vi "Open FPGA Reference.vi"(8 "Error In":errorcluster, 11 "Settings.Compiled":T18={"Name"="", "RIO.Address"="", "Bitfile.Path"=path "", "Injectors.Count"=0, "Injectors.Settings"=[], "Waveform.Refs"=[], "VS.Registers"={"Block Data refs"=[], "Values"=[]}, "Registers"=[], "Timing.Registers"=[], "Mux.Register"={"Name"="", "Data Type"=enum."<Null>", "Default Value"=variant(dbl 0.0)}, "Groups.Settings"=[]} {"Mux.Register"."Data Type" format="%.0x"; "Registers"."Register"."Data Type" format="%.0x"; "VS.Registers"."Block Data refs"."Data Reference" format="%.0x"}) -> (0 "Error Out":errorcluster, 2 "Async Parameters":T1, 3 "Inline State Data out":T13 {"VS.Registers"."Data Reference" format="%.0x"; "FPGA.Registers"."Data Type" format="%.0x"})   [LabVIEW 2019, in "Fuel Injector Analysis Addon Engine.lvlib"]
uses:
  Fuel Injector Analysis Addon Engine.lvlib
  Shared/Types/Compiled.Settings.ctl
  Shared/Types/Injector info.ctl
  Shared/Types/Compiled.Group.WaveformRefs.ctl
  <vilib>/NI VeriStand/Custom Device API/Waveform Data Reference.ctl
  <vilib>/NI VeriStand/Custom Device API/Block Data Reference.ctl
  <vilib>/NI VeriStand/Custom Device API/Data Reference.ctl
  Shared/Types/VS.Register.Info.ctl
  Shared/Types/Register.Info.ctl
  Shared/Types/FPGA Data Types.ctl
  Shared/Types/Compiled.Group.Timing.ctl
  Shared/Types/Shot.Parameters.ctl
  Shared/Types/Stage.Parameters.ctl
  Shared/Types/Stage.PullIn.Types.ctl
  Shared/Types/Stage.Transition.Types.ctl
  Shared/Types/Analysis.Channels.Select.ctl
  Types/Inline State Data.ctl
  <vilib>/NI/NIVS Inline Async API/_VS Inline Async API/VS Inline Async API/VS Inline Async API.lvclass
  Types/FPGA Refs.ctl
  Types/Async Parameters.ctl
  Types/Injector.State.ctl
  <vilib>/NI/NIVS Inline Async API/_Data Access Engine/Data Access Engine/Types/Write.DVR.ctl
  <vilib>/NI/NIVS Inline Async API/_Data Access Engine/Access Type Classes/Write/Write.lvclass
  <vilib>/NI/NIVS Inline Async API/_Data Access Engine/Data Access Engine/Types/Read.DVR.ctl
  <vilib>/NI/NIVS Inline Async API/_Data Access Engine/Access Type Classes/Read/Read.lvclass
  <vilib>/NI VeriStand/Custom Device Waveform API/Single Waveform Write (DBL)/Single Waveform Write (DBL).lvclass
  <vilib>/NI/LVFPGA Adv Session Resources/OpenByNameSubVI.vi
  Shared/Constants.vi
  <vilib>/rvi/interface/common/dynamic/niFpgaEscapeDelimiterAndNull.vi
  <vilib>/Utility/error.llb/Error Cluster From Error Code.vi
  <vilib>/rvi/interface/common/niFpgaWaitOnOcc.vi
  Register.Initialize.vi
  Write To FPGA.vi
  <vilib>/NI/LVFPGA Adv Session Resources/OpenByName.xnode
  <vilib>/rvi/interface/nirviMethod/nirviMethod.xnode
  <vilib>/rvi/errors/niLvFpgaMergeErrorWithErrorCode.vi
  Shared/Fuel Injector Analysis Addon Shared.lvlib
  <vilib>/NI VeriStand/Custom Device API/Custom Device API.lvlib
  <vilib>/FPGAPlugInAG/Dynamic/niLvFpga_ConfigureFifo_Dynamic.vi
  <vilib>/FPGAPlugInAG/Dynamic/niLvFpga_StartFifo_Dynamic.vi
  <vilib>/NI/NIVS Inline Async API/_Data Access Engine/Data Access Engine/Data Access Engine.lvclass
  <vilib>/NI/LVFPGA Adv Session Resources/LVFPGAAdvSessionResources.lvlib
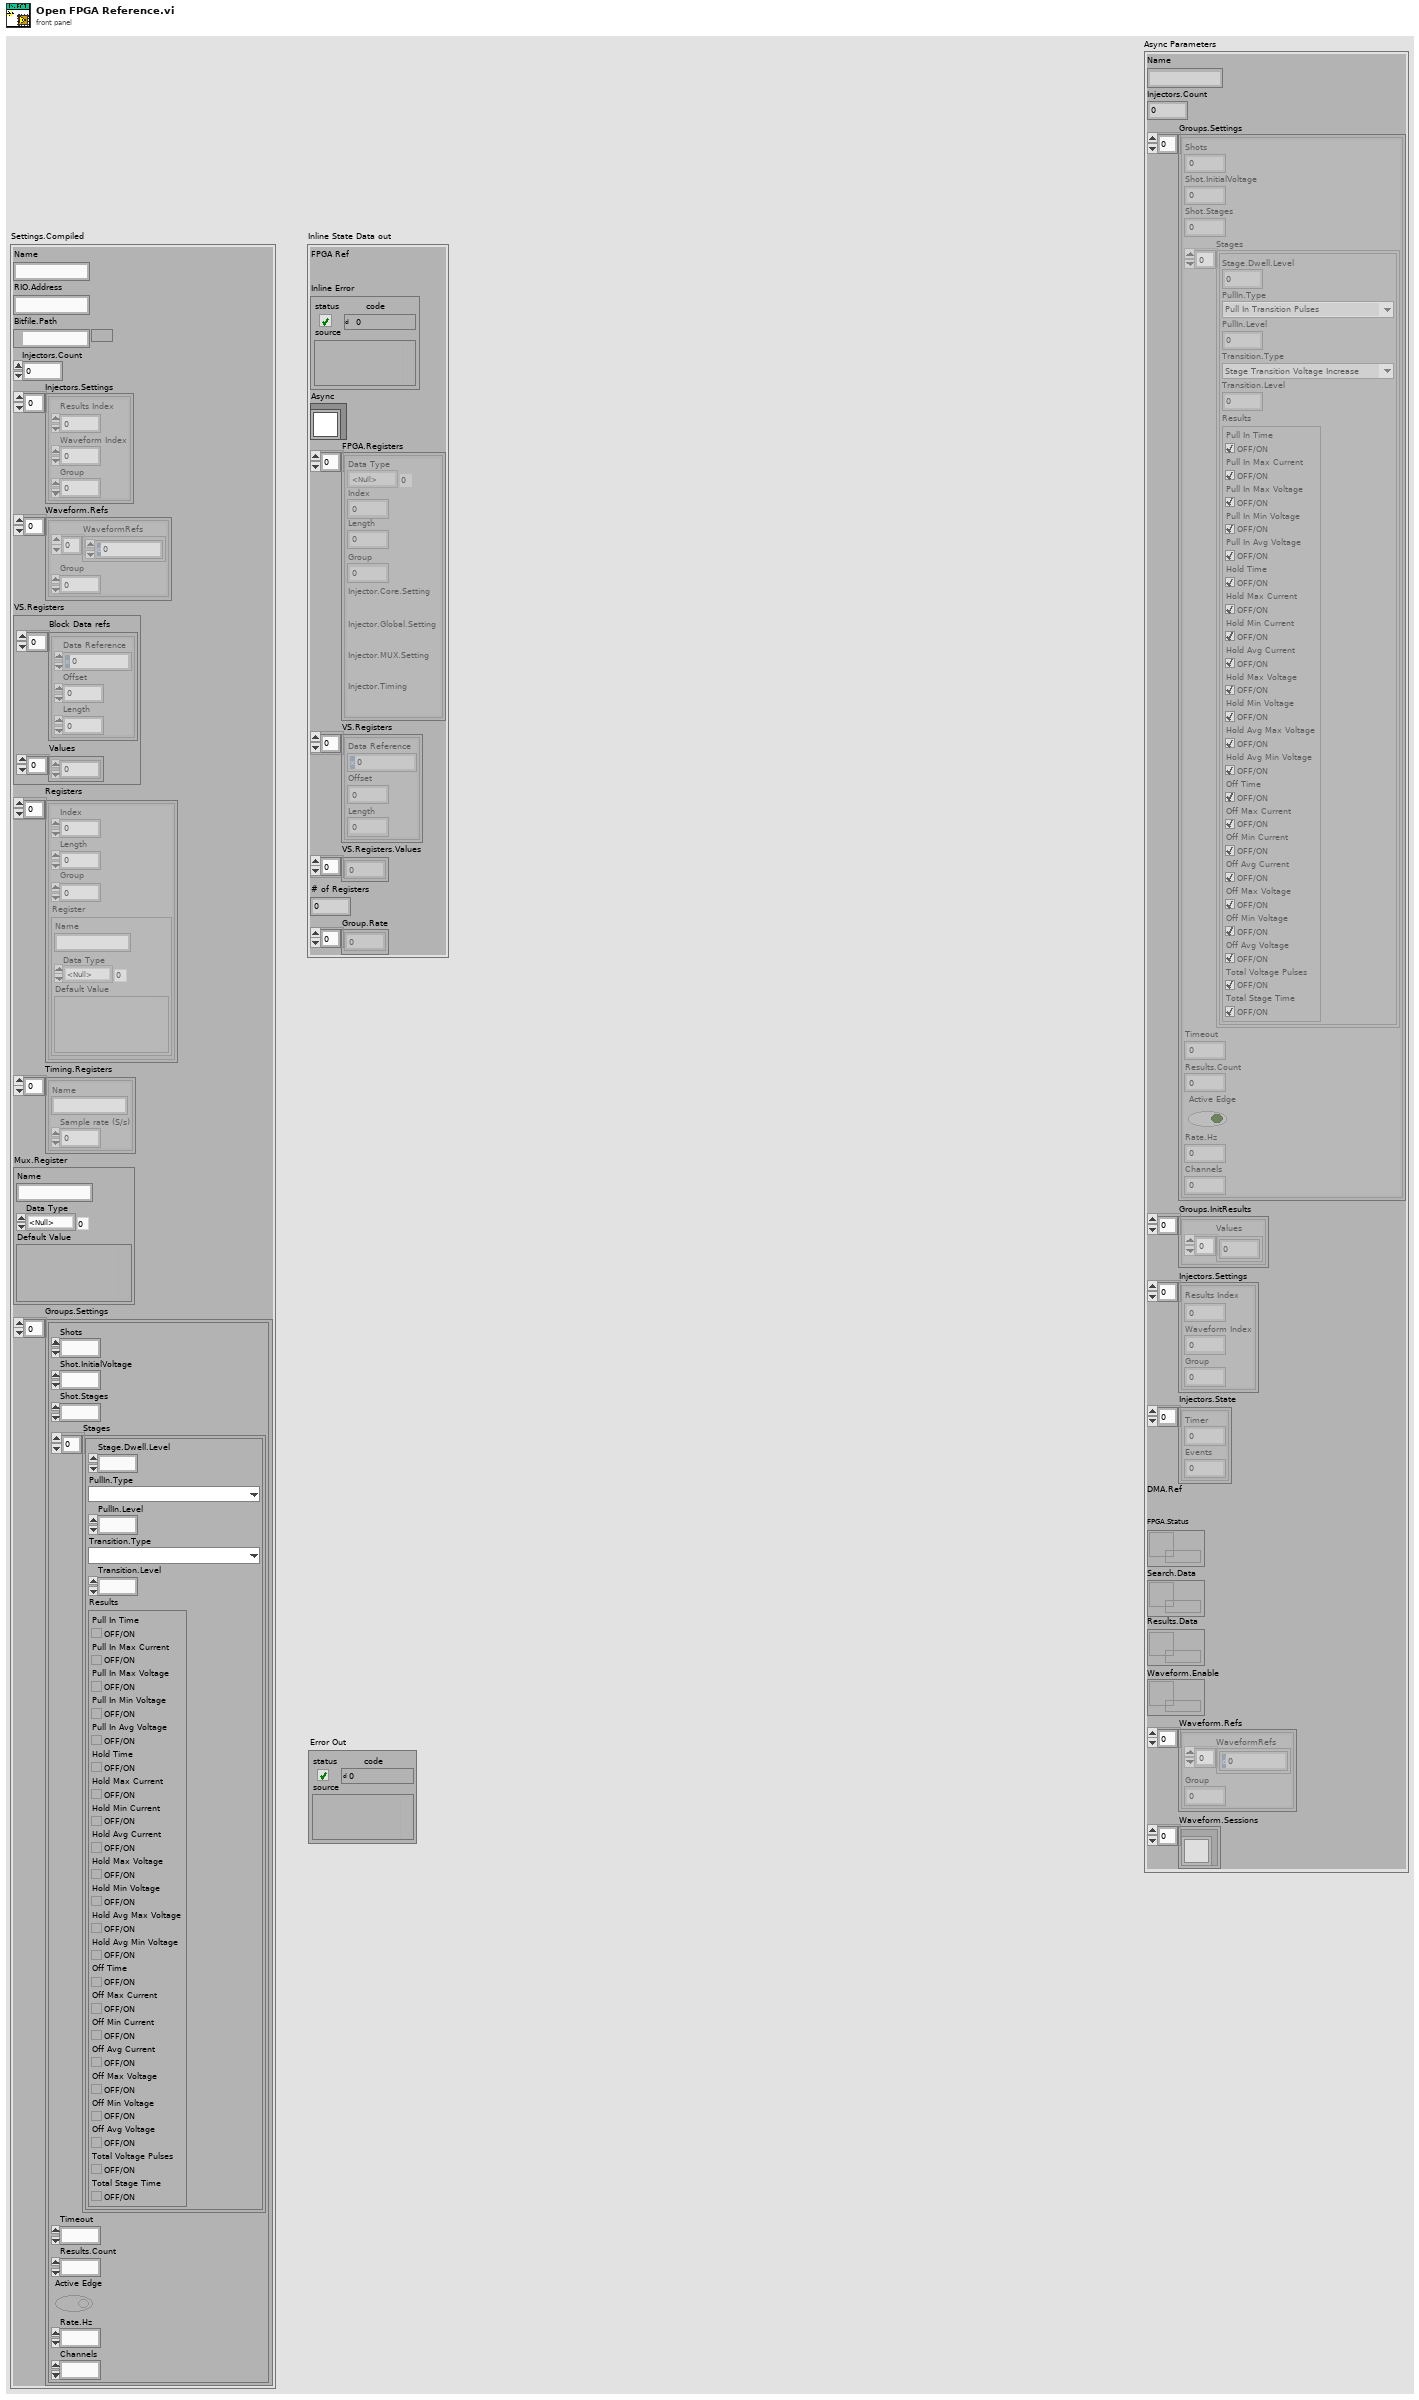
[diagram p1: front panel]
types:
  T1 = typedef "Fuel Injector Analysis Addon Engine.lvlib/Async Parameters.ctl" = cluster{"Name":string, "Injectors.Count":u8, "Groups.Settings":T2[], "Groups.InitResults":cluster{"Values":dbl[]}[], "Injectors.Settings":T7[], "Injectors.State":T8[], "DMA.Ref":refnum<k20>, "FPGA.Status":T9, "Search.Data":T10, "Results.Data":T9, "Waveform.Enable":T10, "Waveform.Refs":T11[], "Waveform.Sessions":refnum<class "Single Waveform Write (DBL).lvclass">[]}
  T2 = typedef "Fuel Injector Analysis Addon Shared.lvlib/Shot.Parameters.ctl" = cluster{"Shots":u32, "Shot.InitialVoltage":dbl, "Shot.Stages":u32, "Stages":T3[], "Timeout":dbl, "Results.Count":i32, "Active Edge":bool, "Rate.Hz":u32, "Channels":u32}
  T3 = typedef "Fuel Injector Analysis Addon Shared.lvlib/Stage.Parameters.ctl" = cluster{"Stage.Dwell.Level":dbl, "PullIn.Type":T4, "PullIn.Level":dbl, "Transition.Type":T5, "Transition.Level":dbl, "Results":T6}
  T4 = typedef "Fuel Injector Analysis Addon Shared.lvlib/Stage.PullIn.Types.ctl" = enum8{"Pull In Transition Pulses", "Pull In Transition Current Drop"}
  T5 = typedef "Fuel Injector Analysis Addon Shared.lvlib/Stage.Transition.Types.ctl" = enum8{"Stage Transition Inactive Time", "Stage Transition Voltage Increase", "Stage Transition Current Decrease", "Stage Transition Active Time"}
  T6 = typedef "Fuel Injector Analysis Addon Shared.lvlib/Analysis.Channels.Select.ctl" = cluster{"Pull In Time":bool, "Pull In Max Current":bool, "Pull In Max Voltage":bool, "Pull In Min Voltage":bool, "Pull In Avg Voltage":bool, "Hold Time":bool, "Hold Max Current":bool, "Hold Min Current":bool, "Hold Avg Current":bool, "Hold Max Voltage":bool, "Hold Min Voltage":bool, "Hold Avg Max Voltage":bool, "Hold Avg Min Voltage":bool, "Off Time":bool, "Off Max Current":bool, "Off Min Current":bool, "Off Avg Current":bool, "Off Max Voltage":bool, "Off Min Voltage":bool, "Off Avg Voltage":bool, "Total Voltage Pulses":bool, "Total Stage Time":bool}
  T7 = typedef "Fuel Injector Analysis Addon Shared.lvlib/Injector info.ctl" = cluster{"Results Index":i32, "Waveform Index":i32, "Group":u16}
  T8 = typedef "Fuel Injector Analysis Addon Engine.lvlib/Injector.State.ctl" = cluster{"Timer":u32, "Events":u64}
  T9 = typedef "Data Access Engine.lvlib/Data Access Engine.lvclass/Write.DVR.ctl" = refnum<data-value>
  T10 = typedef "Data Access Engine.lvlib/Data Access Engine.lvclass/Read.DVR.ctl" = refnum<data-value>
  T11 = typedef "Fuel Injector Analysis Addon Shared.lvlib/Compiled.Group.WaveformRefs.ctl" = cluster{"WaveformRefs":T12[], "Group":i32}
  T12 = typedef "Custom Device API.lvlib/Waveform Data Reference.ctl" = i32
  T13 = typedef "Fuel Injector Analysis Addon Engine.lvlib/Inline State Data.ctl" = cluster{"FPGA Ref":refnum<k20>, "Inline Error":errorcluster, "Async":refnum<class "VS Inline Async API.lvclass">, "FPGA.Registers":T14[], "VS.Registers":T16[], "VS.Registers.Values":dbl[], "# of Registers":u32, "Group.Rate":u32[]}
  T14 = typedef "Fuel Injector Analysis Addon Engine.lvlib/FPGA Refs.ctl" = cluster{"Data Type":T15, "Index":i32, "Length":i32, "Group":i32, "Injector.Core.Setting":refnum<k20>, "Injector.Global.Setting":refnum<k20>, "Injector.MUX.Setting":refnum<k20>, "Injector.Timing":refnum<k20>}
  T15 = typedef "Fuel Injector Analysis Addon Shared.lvlib/FPGA Data Types.ctl" = enum8{"<Null>", "Injector.Core.Setting", "Injector.Global.Setting", "Injector.Mux.Setting", "Injector.Timing"}
  T16 = typedef "Custom Device API.lvlib/Block Data Reference.ctl" = cluster{"Data Reference":T17, "Offset":u64, "Length":u64}
  T17 = typedef "Custom Device API.lvlib/Data Reference.ctl" = i32
  T18 = typedef "Fuel Injector Analysis Addon Shared.lvlib/Compiled.Settings.ctl" = cluster{"Name":string, "RIO.Address":string, "Bitfile.Path":path, "Injectors.Count":u32, "Injectors.Settings":T7[], "Waveform.Refs":T11[], "VS.Registers":cluster{"Block Data refs":T16[], "Values":dbl[]}, "Registers":T19[], "Timing.Registers":T21[], "Mux.Register":T20, "Groups.Settings":T2[]}
  T19 = typedef "Fuel Injector Analysis Addon Shared.lvlib/VS.Register.Info.ctl" = cluster{"Index":i32, "Length":i32, "Group":i32, "Register":T20}
  T20 = typedef "Fuel Injector Analysis Addon Shared.lvlib/Register.Info.ctl" = cluster{"Name":string, "Data Type":T15, "Default Value":variant}
  T21 = typedef "Fuel Injector Analysis Addon Shared.lvlib/Compiled.Group.Timing.ctl" = cluster{"Name":string, "Sample rate (S/s)":u32}
  T22 = cluster{"Name":string, "Depth":u32, "Write? (Deprecated:Use Implementation)":bool, "Physical Channel":u32, "Base Address":u32, "Data Width":u32, "Data Type":enum32{"Boolean", "I8", "I16", "I32", "I64", "U8", "U16", "U32", "U64", "FXP", "CustomControl", "SGL"}, "FXP Properties":variant, "Write Window Address":u32, "Implementation":enum16{"niFpgaTargetToHost", "niFpgaHostToTarget", "niFpgaPeerToPeerWriter", "niFpgaPeerToPeerReader", "niCoreTargetToHost", "niCoreHostToTarget"}, "Control Set":u32}[]
  T23 = cluster{"Name":string, "type":variant, "indicator?":bool}[]
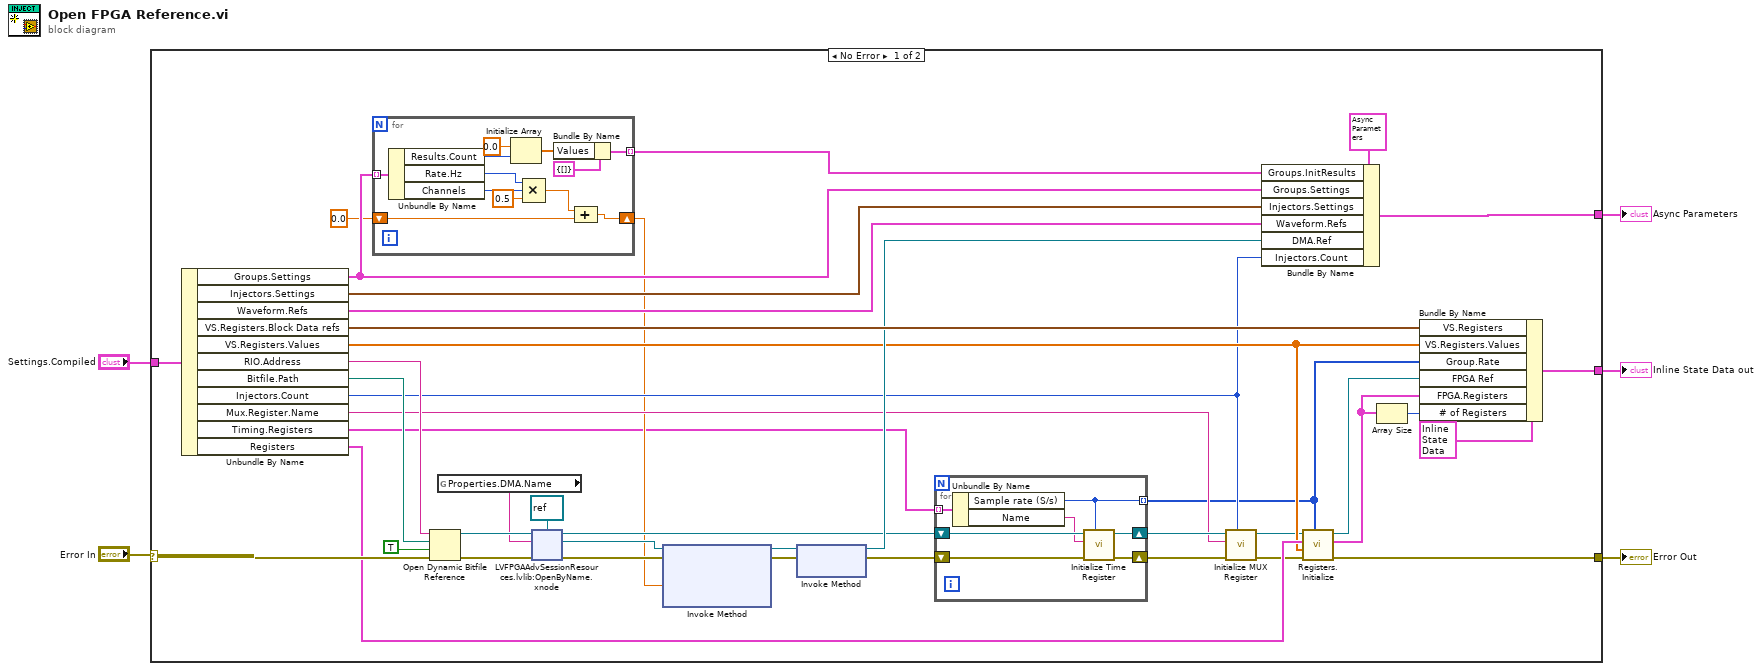
[diagram p0: block diagram]
diagram:
  n1 = case shown="No Error" "Error In" {
    selector: "Error In" -> [w45 w79]
    tunnel: [w34 w79] -> w4
    tunnel: "Settings.Compiled" -> [w29 _]
    tunnel: [w30 _] -> w2
    tunnel: [w23 _] -> w1
    frame No Error {
      n2 = Unbundle By Name(w29) -> ("Groups.Settings"=w12:T2[], "Injectors.Settings"=w25:T7[], "Waveform.Refs"=w26:T11[], "VS.Registers.Block Data refs"=w28:T16[], "VS.Registers.Values"=w18:dbl[], "RIO.Address"=w43:string, "Bitfile.Path"=w44:path, "Injectors.Count"=w10:u32, "Mux.Register.Name"=w13:string, "Timing.Registers"=w7:T21[], "Registers"=w33:T19[])
      n3 = for {
        tunnel: [w60] -> w11 mode=indexing
        tunnel: w12 -> [w64] mode=indexing
        shift-right: [w55] -> w8
        shift-left: 0.0 -> [w54]
        n4 = Unbundle By Name(w64) -> ("Results.Count"=w63:i32, "Rate.Hz"=w58:u32, "Channels"=w57:u32)
        n5 = Initialize Array(0.0, w63) -> (w61:dbl[])
        n6 = Compound Arithmetic op=MULTIPLY(w58, w57, 0.5 ("value")) -> (w56:dbl)
        n7 = Bundle By Name(cluster=cluster{"Values":dbl[]} {"Values"=[]} ("Values"), "Values"=w61) -> (w60:cluster{"Values":dbl[]})
        n8 = Compound Arithmetic op=ADD(w56, w54) -> (w55:dbl)
      }
      n9 = Open Dynamic Bitfile Reference(0:w43, 1:w44, 2:TRUE ("Run When Loaded"), 3:w45) -> (5:w36:refnum<k20>, 8:w37:errorcluster)  [unwired: 1 in]
      n10 = global read "Constants.vi" "Properties.DMA.Name"() -> (w35:string)
      n11 = xnode "LVFPGAAdvSessionResources.lvlib:OpenByName.xnode"("FPGA VI Reference in"=w36, "Resource name in"=w35, "Single resource reference type in"=refnum<k20> refnum, "Error in"=w37) -> ("Single resource reference out"=w38:refnum<k20>, "Error out"=w39:errorcluster, "FPGA VI Reference out"=w19:refnum<k20>)
      n12 = xnode "Invoke Method"("FPGA VI Reference In"=w38, "error in"=w39, "Requested Depth"=w8) -> ("FPGA VI Reference Out"=w41:refnum<k20>, "error out"=w40:errorcluster)  [unwired: 1 out]
      n13 = xnode "Invoke Method"("FPGA VI Reference In"=w41, "error in"=w40) -> ("FPGA VI Reference Out"=w27:refnum<k20>, "error out"=w20:errorcluster)
      n14 = for {
        shift-right: [w51] -> w17
        shift-left: w20 -> [w53]
        shift-right: [w50] -> w14
        shift-left: w19 -> [w52]
        tunnel: w7 -> [w49] mode=indexing
        tunnel: [w47] -> w6 mode=indexing
        n15 = Unbundle By Name(w49) -> ("Sample rate (S/s)"=w47:u32, "Name"=w48:string)
        n16 = call "Initialize Time Register.vi"("Sample rate (Hz)"=w47, "error in (no error)"=w53, "Name"=w48, "FPGA Ref"=w52) -> ("error out"=w51:errorcluster, "FPGA Ref out"=w50:refnum<k20>)  [unwired: 6 in]
      }
      n17 = call "Initialize MUX Register.vi"("# of Injectors"=w10, "error in (no error)"=w17, "Name"=w13, "FPGA Ref"=w14) -> ("error out"=w16:errorcluster, "FPGA Ref out"=w15:refnum<k20>)  [unwired: 6 in]
      n18 = Bundle By Name(cluster=T1 {"Name"="", "Injectors.Count"=0, "Groups.Settings"=[], "Groups.InitResults"=[], "Injectors.Settings"=[], "Injectors.State"=[], "DMA.Ref"=refnum, "FPGA.Status"=refnum, "Search.Data"=refnum, "Results.Data"=refnum, "Waveform.Enable"=refnum, "Waveform.Refs"=[], "Waveform.Sessions"=[]} ("Async Parameters"), "Groups.InitResults"=w11, "Groups.Settings"=w12, "Injectors.Settings"=w25, "Waveform.Refs"=w26, "DMA.Ref"=w27, "Injectors.Count"=w10) -> (w23:T1)
      n19 = call "Registers.Initialize.vi"("Group.Rate"=w6, "error in (no error)"=w16, "Values"=w18, "Registers"=w33, "FPGA Ref"=w15) -> ("error out"=w34:errorcluster, "Registers Ref"=w22:T14[], "FPGA Ref out"=w24:refnum<k20>)  [unwired: 4 in]
      n20 = Array Size(array=w22) -> (size(s)=w21:i32)
      n21 = Bundle By Name(cluster=T13 {"FPGA Ref"=refnum, "Inline Error"={"status"=FALSE, "code"=0, "source"=""}, "Async"=refnum, "FPGA.Registers"=[], "VS.Registers"=[], "VS.Registers.Values"=[], "# of Registers"=0, "Group.Rate"=[]} ("Inline State Data out"), "VS.Registers"=w28, "VS.Registers.Values"=w18, "Group.Rate"=w6, "FPGA Ref"=w24, "FPGA.Registers"=w22, "# of Registers"=w21) -> (w30:T13)
    }
    frame Error {
    }
  }
  "Error Out" <- w4
  "Inline State Data out" <- w2
  "Async Parameters" <- w1
